vi "Recurse.vi"(9 "Depth":u32, 10 "State":map{u32, string}(c390), 11 "Input":string) -> (1 "State 2":map{u32, string}(c390), 2 "Complexity":u64)   [LabVIEW 2020]
uses:
  Memory Global.vi
  Directional Keypad/Directional Keypad.lvclass
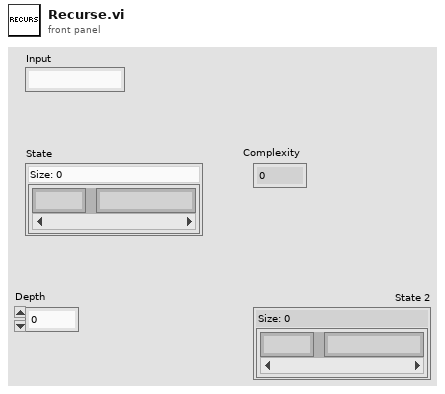
[diagram p1: front panel]
types:
  T1 = map{cluster{"Input":string, "Depth":u32, "Current position":string}, cluster{"default value":u64, "default value":string}}
  T2 = cluster{"default value":u64, "default value":string}
  T3 = cluster{"Input":string, "Depth":u32, "Current position":string}
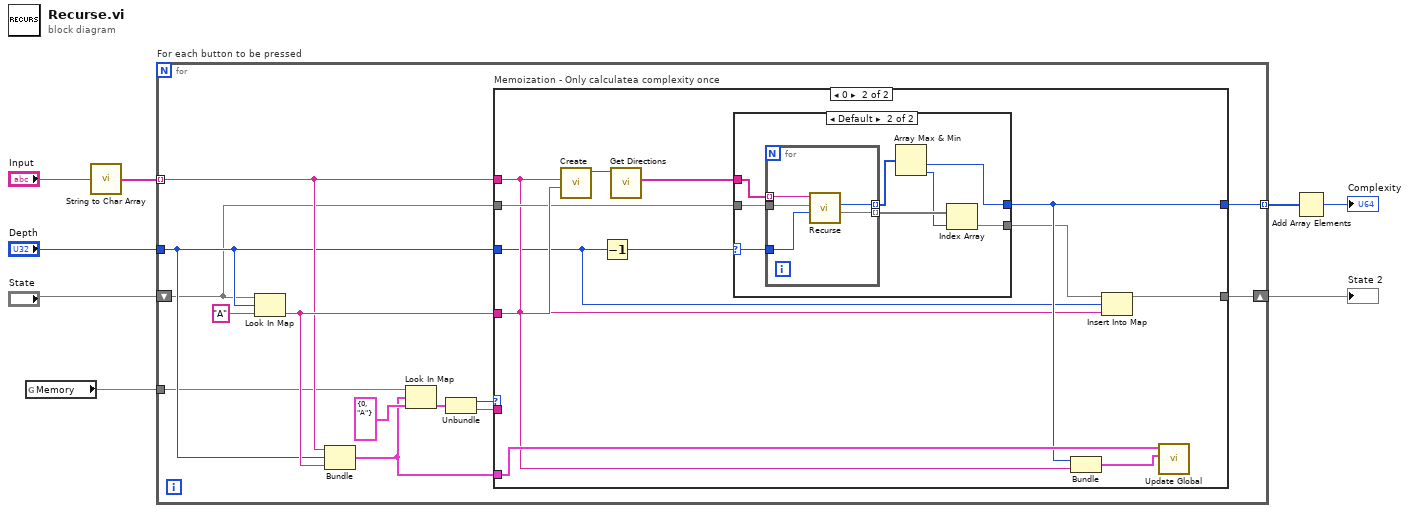
[diagram p0: block diagram]
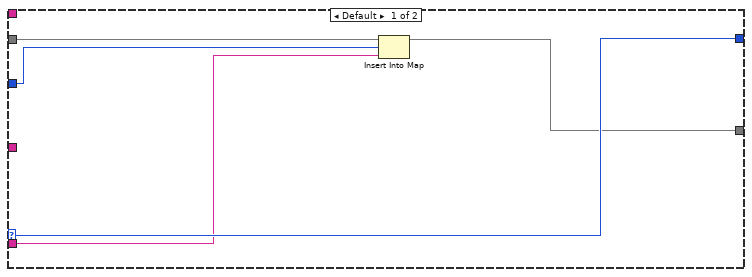
[diagram p2: hidden frame]
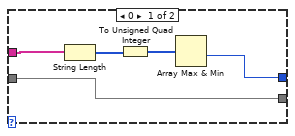
[diagram p3: hidden frame]
diagram:
  n1 = global read "Memory Global.vi" "Memory"() -> (w1:T1)
  n2 = call "String to Char Array.vi"("Input"="Input") -> ("Array"=w5:string[])
  n3 = for "For each button to be pressed" {
    tunnel: "Depth" -> [w12]
    tunnel: [w21] -> w7 mode=indexing
    tunnel: w5 -> [w13] mode=indexing
    shift-right: [w19] -> w3
    shift-left: "State" -> [w11]
    tunnel: w1 -> [w10]
    n4 = Look In Map(map=w11, key=w12, default value="A") -> (value=w17:string)  [unwired: 1 out]
    n5 = Bundle("Input"=w13, "Depth"=w12, "Current position"=w17) -> (w14:T3)  [unwired: 1 in]
    n6 = Look In Map(map=w10, key=w14, default value=T2 {"default value"=0, "default value"="A"}) -> (value=w18:T2)  [unwired: 1 out]
    n7 = Unbundle(w18) -> ("default value"=w9:u64, "default value"=w15:string)
    n8 = case "Memoization - Only calculatea complexity once" shown="0" w9 {
      selector: w9 -> [w26 _]
      tunnel: [w26 w35] -> w21
      tunnel: w12 -> [w22 w27]
      tunnel: w11 -> [w25 w32]
      tunnel: [w24 w30] -> w19
      tunnel: w13 -> [_ w29]
      tunnel: w17 -> [_ w33]
      tunnel: w14 -> [_ w36]
      tunnel: w15 -> [w23 _]
      frame Default {
        n9 = Insert Into Map(map in=w25, key=w22, value=w23) -> (map out=w24:map{u32, string})  [unwired: 2 out]
      }
      frame 0 {
        n10 = call "Create.vi"("Current"=w33, "Input"=w29) -> ("Proto"=w38:refnum<class "Directional Keypad.lvclass">)  [unwired: 9 in]
        n11 = Decrement(x=w27) -> (x-1=w28:u32)
        n12 = call "Get Directions.vi"("Proto in"=w38) -> ("Directional Button Presses"=w37:string[])  [unwired: 9 in, 1 out]
        n13 = case shown="Default" w28 {
          selector: w28 -> [_ w51]
          tunnel: w37 -> [w41 w50]
          tunnel: [w39 w45] -> w35
          tunnel: [w42 w47] -> w31
          tunnel: w32 -> [w42 w48]
          frame 0 {
            n14 = String Length(string=w41) -> (length=w40:i32[])
            n15 = To Unsigned Quad Integer(1:w40) -> (0:w43:u64[])
            n16 = Array Max & Min(array=w43) -> (min value=w39:u64)  [unwired: 3 out]
          }
          frame Default {
            n17 = for {
              tunnel: w51 -> [w56]
              tunnel: [w55] -> w46 mode=indexing
              tunnel: w50 -> [w54] mode=indexing
              tunnel: [w53] -> w49 mode=indexing
              tunnel: w48 -> [w52]
              n18 = call "Recurse.vi"("Depth"=w56, "State"=w52, "Input"=w54) -> ("State 2"=w53:map{u32, string}, "Complexity"=w55:u64)  [unwired: 7 in]
            }
            n19 = Array Max & Min(array=w46) -> (min value=w45:u64, min index (indices)=w44:i32)  [unwired: 2 out]
            n20 = Index Array(array=w49, index=w44) -> (element=w47:map{u32, string})
          }
        }
        n21 = Bundle(w35, "Input"=w29) -> (w34:cluster{u64, "Input":string})  [unwired: 1 in]
        n22 = Insert Into Map(map in=w31, key=w27, value=w29) -> (map out=w30:map{u32, string})  [unwired: 2 out]
        n23 = call "Update Global.vi"("Val"=w34, "Key"=w36) -> ()  [unwired: 10 in]
      }
    }
  }
  "State 2" <- w3
  n24 = Add Array Elements(numeric array=w7) -> (sum=→"Complexity":u64)
